vi "Global_SM Write_Data Out.vi"() -> ()   [LabVIEW 2017, in "Gimbal.lvlib"]
uses:
  startup.rtexe/Gimbal.lvlib
panel:
  in  "Gimbal_SM_UpDownAngleSet":i32(slide) scale=-90.0..90.0
  in  "Gimbal_SM_LeftRightAngleSet":i32(slide) scale=-90.0..90.0
  # "The Names of the Data items in the Global Variable MUST describe who the Single Writer is\nNaming Convention of all Data Items is:   \nLib Name_Loop Name (SM or SEN or ACT)_Data Name\nExamples:\nDrive_ACT_X axis\nGameController_SEN_JoystickLeft\nHopper_SM_AgitatorSpeed"
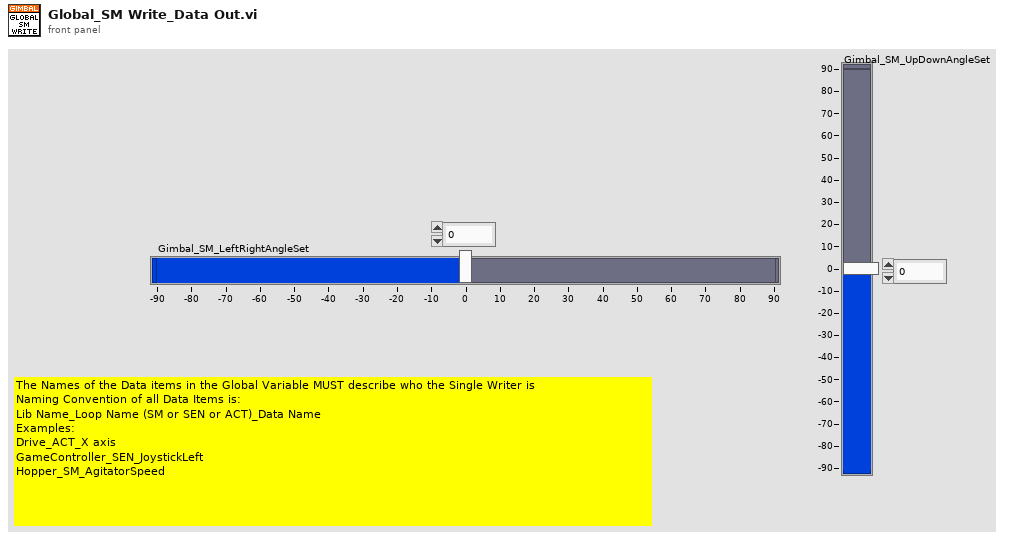
[diagram p1: front panel]
diagram:
